vi "port to indices.vi"(11 "Port":cluster{"module":u8, "channel":u8}[](array[cluster])) -> (3 "Channel Indices":i32[](array[numeric]))   [LabVIEW 2012]
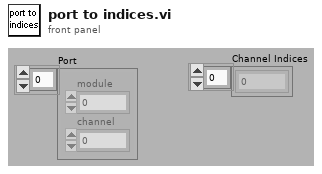
[diagram p1: front panel]
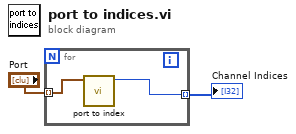
[diagram p0: block diagram]
diagram:
  n1 = for {
    tunnel: [w3] -> w2 mode=indexing
    tunnel: "Port" -> [w4] mode=indexing
    n2 = call "port to index.vi"("Port"=w4) -> ("Channel Index"=w3:i32)  [unwired: 10 in]
  }
  "Channel Indices" <- w2
